vi "CRYLimit Table Delete Item.vi"(9 "Selection Size":T1, 10 "Selection Start":T1, 11 "Table In":string[][](array[string])) -> (3 "Table Out":string[][](array[string]))   [LabVIEW 2013]
uses:
  <vilib>/Utility/miscctls.llb/LVRowAndColumnTypeDef.ctl
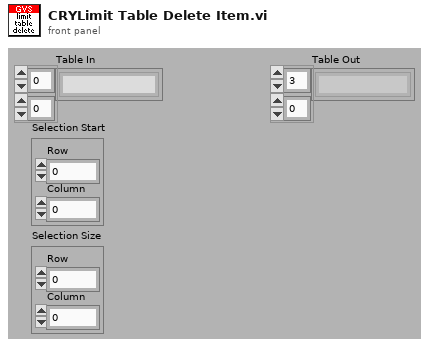
[diagram p1: front panel]
types:
  T1 = typedef "LVRowAndColumnTypeDef.ctl" = cluster{"Row":i32, "Column":i32}
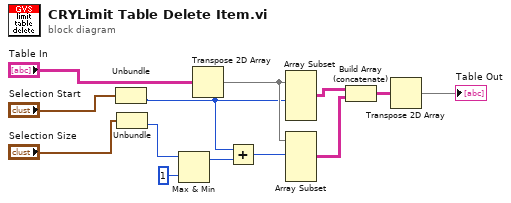
[diagram p0: block diagram]
diagram:
  n1 = Unbundle("Selection Start") -> ("Column"=w6:i32)  [unwired: 1 out]
  n2 = Unbundle("Selection Size") -> ("Column"=w5:i32)  [unwired: 1 out]
  n3 = Max & Min(x=w5, y=1 ("Number of columns")) -> (max(x,y)=w7:i32)  [unwired: 1 out]
  n4 = Transpose 2D Array(2D array="Table In") -> (transposed array=w13:string[][])
  n5 = Add(x=w6, y=w7) -> (x+y=w9:i32)
  n6 = Array Subset(array=w13, length (row)=w6) -> (w12:string[][])  [unwired: 3 in]
  n7 = Array Subset(array=w13, index (row)=w9) -> (w11:string[][])  [unwired: 3 in]
  n8 = Build Array (concatenate)(w12, w11) -> (w10:string[][])
  n9 = Transpose 2D Array(2D array=w10) -> (transposed array=→"Table Out":string[][])
